vi "split.vi"(0 "object in":refnum<class "interface.lvclass">, 1 "输入数据":string[][](array[string]), 2 "拆分大小":i32=1000, 5 "error in (no error)":errorcluster) -> (14 "object out":refnum<class "interface.lvclass">, 15 "输出数组":string[][](array[string]), 16 "拆分数据":bool, 19 "error out":errorcluster)   [LabVIEW 2016, in "interface.lvclass"]
uses:
  interface.lvclass
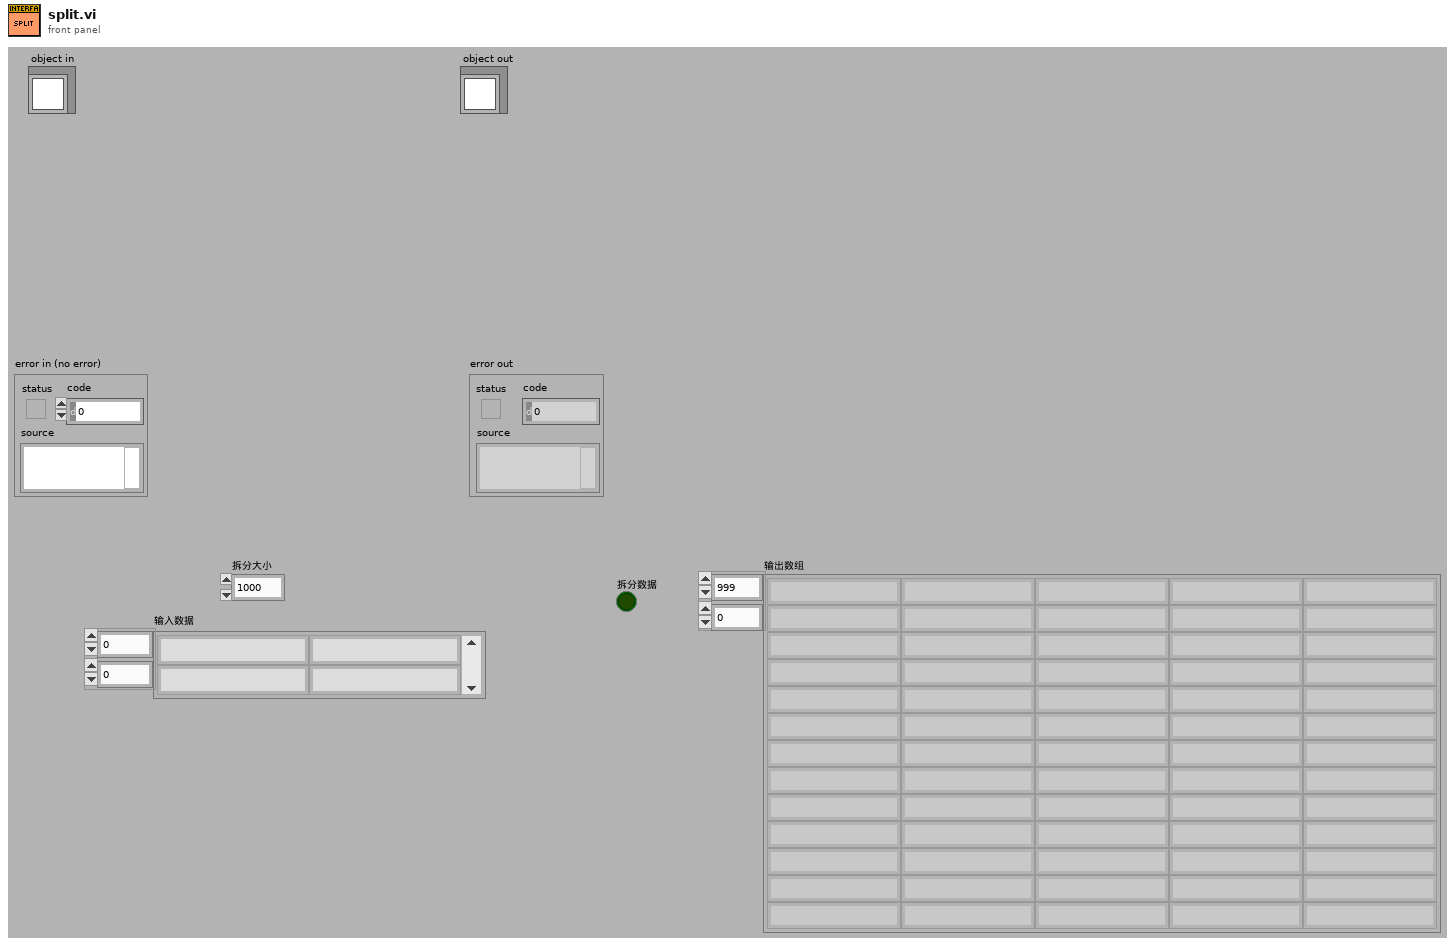
[diagram p1: front panel]
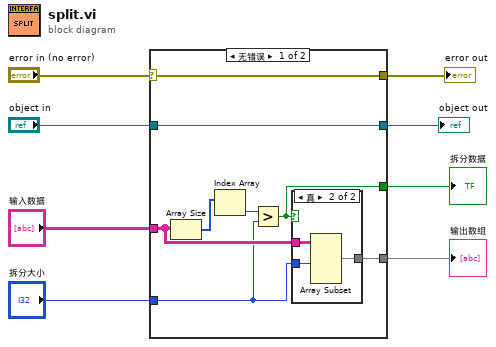
[diagram p0: block diagram]
diagram:
  n1 = case shown="无错误" "error in (no error)" {
    selector: "error in (no error)" -> [w16 w22]
    tunnel: [w16 w22] -> w7
    tunnel: [w15 w21] -> w5
    tunnel: "object in" -> [w15 w21]
    tunnel: "输入数据" -> [w12 _]
    tunnel: "拆分大小" -> [w11 _]
    tunnel: [w10 _] -> w2
    tunnel: [w9 _] -> w1
    frame No Error {
      n2 = Array Size(array=w12) -> (size(s)=w14:i32[])
      n3 = Index Array(array=w14) -> (element=w13:i32)  [unwired: 1 in]
      n4 = Greater?(x=w13, y=w11) -> (0:w10:bool)
      n5 = case shown="真" w10 {
        tunnel: w12 -> [w17 w20]
        tunnel: w11 -> [_ w19]
        tunnel: [w17 w18] -> w9
        frame False {
        }
        frame True {
          n6 = Array Subset(array=w20, length (row)=w19) -> (w18:string[][])  [unwired: 3 in]
        }
      }
    }
    frame Error {
    }
  }
  "error out" <- w7
  "object out" <- w5
  "输出数组" <- w1
  "拆分数据" <- w2
